vi "控件位置读取.vi"(8 "错误输入（无错误）":errorcluster, 11 "控件引用输入":refnum<vi>) -> (0 "错误输出":errorcluster, 2 "位置":T1, 3 "引用输出":refnum<vi>)   [LabVIEW 8.6, in "窗口操作.lvlib"]
uses:
  <vilib>/Utility/miscctls.llb/LVPositionTypeDef.ctl
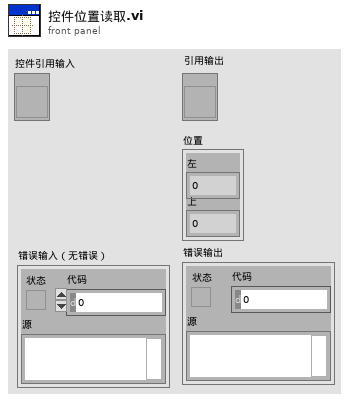
[diagram p1: front panel]
types:
  T1 = typedef "LVPositionTypeDef.ctl" = cluster{"Left":i32, "Top":i32}
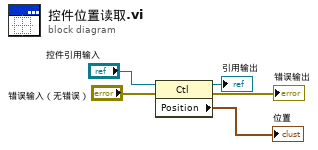
[diagram p0: block diagram]
diagram:
  n1 = property on="Property Node" class="Ctl"(reference="控件引用输入", error in="错误输入（无错误）") -> (reference out=→"引用输出":refnum<vi>, error out=→"错误输出":errorcluster, "Position"=→"位置":T1)
